vi "Is Target Clipped.vi"(8 "Image Size":cluster{i32, i32}, 11 "Bounding Box":T2) -> (3 "Clipped Edge":T1)   [LabVIEW 2011]
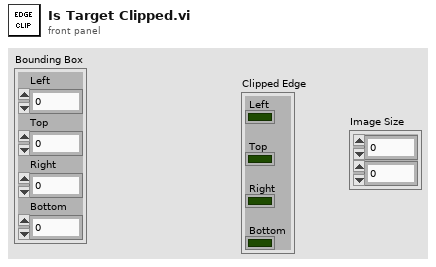
[diagram p1: front panel]
types:
  T1 = cluster{"Left":bool, "Top":bool, "Right":bool, "Bottom":bool}
  T2 = cluster{"Left":dbl, "Top":dbl, "Right":dbl, "Bottom":dbl}
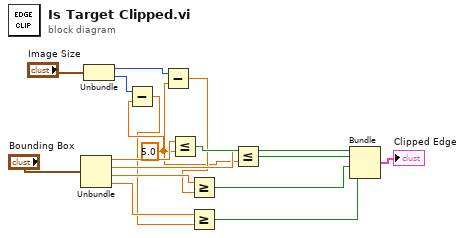
[diagram p0: block diagram]
diagram:
  w2 = 5.0 ("y")
  n1 = Unbundle("Bounding Box") -> ("Left"=w14:dbl, "Top"=w11:dbl, "Right"=w10:dbl, "Bottom"=w8:dbl)
  n2 = Unbundle("Image Size") -> (w5:i32, w3:i32)
  n3 = Subtract(x=w3, y=w2) -> (x-y=w1:dbl)
  n4 = Subtract(x=w5, y=w2) -> (x-y=w4:dbl)
  n5 = Less Or Equal?(x=w14, y=w2) -> (x <= y?=w13:bool)
  n6 = Greater Or Equal?(x=w10, y=w4) -> (x >= y?=w9:bool)
  n7 = Greater Or Equal?(x=w8, y=w1) -> (x >= y?=w7:bool)
  n8 = Less Or Equal?(x=w11, y=w2) -> (x <= y?=w12:bool)
  n9 = Bundle(w13, w12, w9, w7) -> (→"Clipped Edge":cluster{bool, bool, bool, bool})  [unwired: 1 in]
